vi "TCP Read from Connection.vi"(5 "Options":T1={"Ignore Timeout Error"=TRUE, "timeout ms (1000)"=1000}, 7 "error in":errorcluster, 8 "index":i32) -> (0 "error out":errorcluster, 1 "Name":T2, 2 "data string":string, 4 "Timed Out?":bool)   [LabVIEW 2013]
doc: "This VI reads an incoming package of data from the connection specified by \"index\". This VI parses the package and extracts the data name and type as described in the meta data.\n\nFor the package to be parsed correctly, the meta data must be consistent in both the sender and the receiver. The data is packaged based on the existing meta data on the sender."
uses:
  stm_MetaDataElement.ctl
  stm_TCP Read Options.ctl
  Connection Manager/TCP/TCP Connection Method.ctl
  NI STM.lvlib
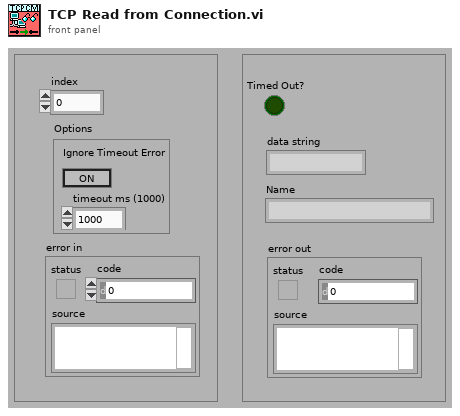
[diagram p1: front panel]
types:
  T1 = typedef "stm_TCP Read Options.ctl" = cluster{"Ignore Timeout Error":bool, "timeout ms (1000)":i32}
  T2 = typedef "stm_MetaDataElement.ctl" = string
  T3 = typedef "NI STM.lvlib/TCP Connection Method.ctl" = enum16{"Initialize", "Add Connection", "Set Properties", "Get Connection(s)", "Remove Connection", "Remove All Connections", "Get Connection Count"}
  T4 = typedef "NI STM.lvlib/TCP Connection Info.ctl" = cluster{"connection ID":refnum<k5>, "meta data":T5[]}
  T5 = typedef "NI STM.lvlib/MetaDataElement.ctl" = string
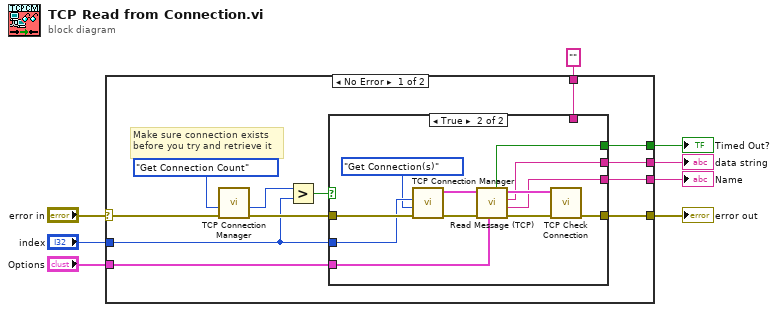
[diagram p0: block diagram]
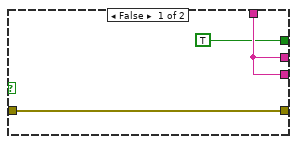
[diagram p2: hidden frame]
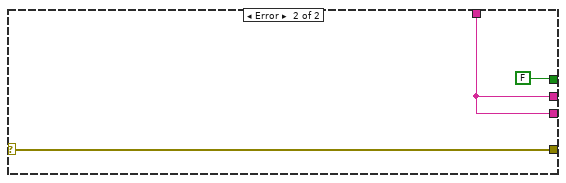
[diagram p3: hidden frame]
diagram:
  n1 = case shown="No Error" "error in" {
    selector: "error in" -> [w18 w38]
    tunnel: [w20 w38] -> w8
    tunnel: [w17 FALSE ("Timed Out?")] -> w6
    tunnel: [w16 w37] -> w5
    tunnel: [w15 w37] -> w4
    tunnel: "" ("data string") -> [w14 w37]
    tunnel: "Options" -> [w13 _]
    tunnel: "index" -> [w11 _]
    frame No Error {
      # "Make sure connection exists\nbefore you try and retrieve it"
      n2 = call "TCP Connection Manager.vi"("error in"=w18, "method"=TCP_Connection_Method."Get Connection Count" ("Method")) -> ("error out"=w19:errorcluster, "number of connections"=w12:i32)  [unwired: 4 in, 4 out]
      n3 = Greater?(x=w12, y=w11) -> (0:w10:bool)
      n4 = case shown="True" w10 {
        tunnel: w19 -> [w23 w28]
        tunnel: [w23 w35] -> w20
        tunnel: [TRUE ("Timed Out?") w32] -> w17
        tunnel: [w22 w31] -> w16
        tunnel: [w22 w30] -> w15
        tunnel: w14 -> [w22 _]
        tunnel: w13 -> [_ w29]
        tunnel: w11 -> [_ w25]
        frame False {
        }
        frame True {
          n5 = call "TCP Connection Manager.vi"("error in"=w28, "method"=TCP_Connection_Method."Get Connection(s)" ("Method"), "index"=w25) -> ("error out"=w27:errorcluster, "connection out"=w26:T4)  [unwired: 3 in, 4 out]
          n6 = call "Read Message (TCP).vi"("options"=w29, "error in"=w27, "connection info in"=w26) -> ("error out"=w33:errorcluster, "name"=w30:T5, "data string"=w31:string, "connection info out"=w34:T4, "timed out?"=w32:bool)  [unwired: 3 in, 1 out]
          n7 = call "TCP Check Connection.vi"("error in"=w33, "connection in"=w34) -> ("error out"=w35:errorcluster)  [unwired: 7 in, 2 out]
        }
      }
    }
    frame Error {
    }
  }
  "error out" <- w8
  "Timed Out?" <- w6
  "data string" <- w5
  "Name" <- w4
